vi "robust-battery-agent.vi"() -> ()   [LabVIEW 2021]
uses:
  General purpose/MEAS.ctl
  General purpose/REQ.ctl
  General purpose/agent-variables.ctl
  General purpose/daemon-config.ctl
panel:
  in  "daemon-config":T1={"resource-type"="battery", "agent-id"=12, "GA-ip"="192.168.1.1", "GA-port"=52020, "RA-ip"="127.0.0.1", "RA-port"=52001, "listenport-RA-side"=52011, "listenport-GA-side"=52021, "local-ip"="192.168.1.12", "long-term"=FALSE}
  in  "param":T2={"Srated"=25000.0, "eta [pu]"=0.98, "model"={"in-states"={"v1"=0.0, "v2"=0.0, "SoC"=0.0}, "output"={"V"=0.0, "Zeq"=0.0, "Eeq"=0.0}}} {"model"."output"."Eeq" format="%#.6g"; "model"."output"."Zeq" format="%#.6g"; "eta [pu]" format="%#_13g"}
  out "json-adv":string
  out "error out":errorcluster
  in  "ra-res config":T3={"resource-type"="battery", "res-ip"="127.0.0.1", "write-port"=32001, "listen-port"=32011}
  out "wake-up":timestamp
  out "uc":cluster{"Pc":dbl, "Qc":dbl}
  in  "model-dt":u32=100
  in  "SoC_T":dbl=50.0
  out "REQ":T4
  in  "main stop":bool
  out "Meas":T5 {"Ud" format="%#.2f"; "P" format="%#.2f"; "Q" format="%#.2f"}
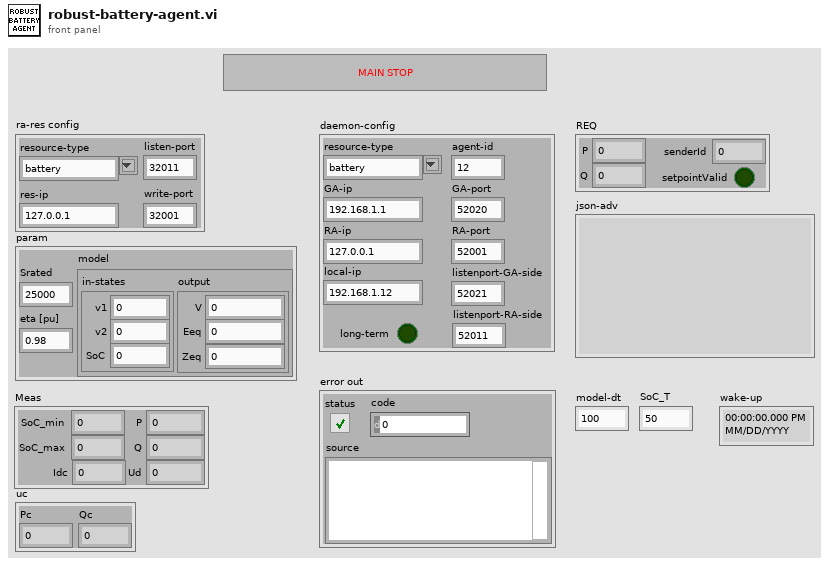
[diagram p1: front panel]
types:
  T1 = typedef "daemon-config.ctl" = cluster{"resource-type":string, "agent-id":u16, "GA-ip":string, "GA-port":u16, "RA-ip":string, "RA-port":u16, "listenport-RA-side":u16, "listenport-GA-side":u16, "local-ip":string, "long-term":bool}
  T2 = typedef "agent-variables.ctl" = cluster{"Srated":dbl, "eta [pu]":dbl, "model":cluster{"in-states":cluster{"v1":dbl, "v2":dbl, "SoC":dbl}, "output":cluster{"V":dbl, "Zeq":dbl, "Eeq":dbl}}}
  T3 = cluster{"resource-type":string, "res-ip":string, "write-port":u16, "listen-port":u16}
  T4 = typedef "REQ.ctl" = cluster{"P":dbl, "Q":dbl, "senderId":u32, "setpointValid":bool}
  T5 = typedef "MEAS.ctl" = cluster{"P":dbl, "Q":dbl, "SoC_max":dbl, "SoC_min":dbl, "Ud":dbl, "Idc":dbl}
  T6 = cluster{"in-states":cluster{"v1":dbl, "v2":dbl, "SoC":dbl}, "output":cluster{"V":dbl, "Zeq":dbl, "Eeq":dbl}}
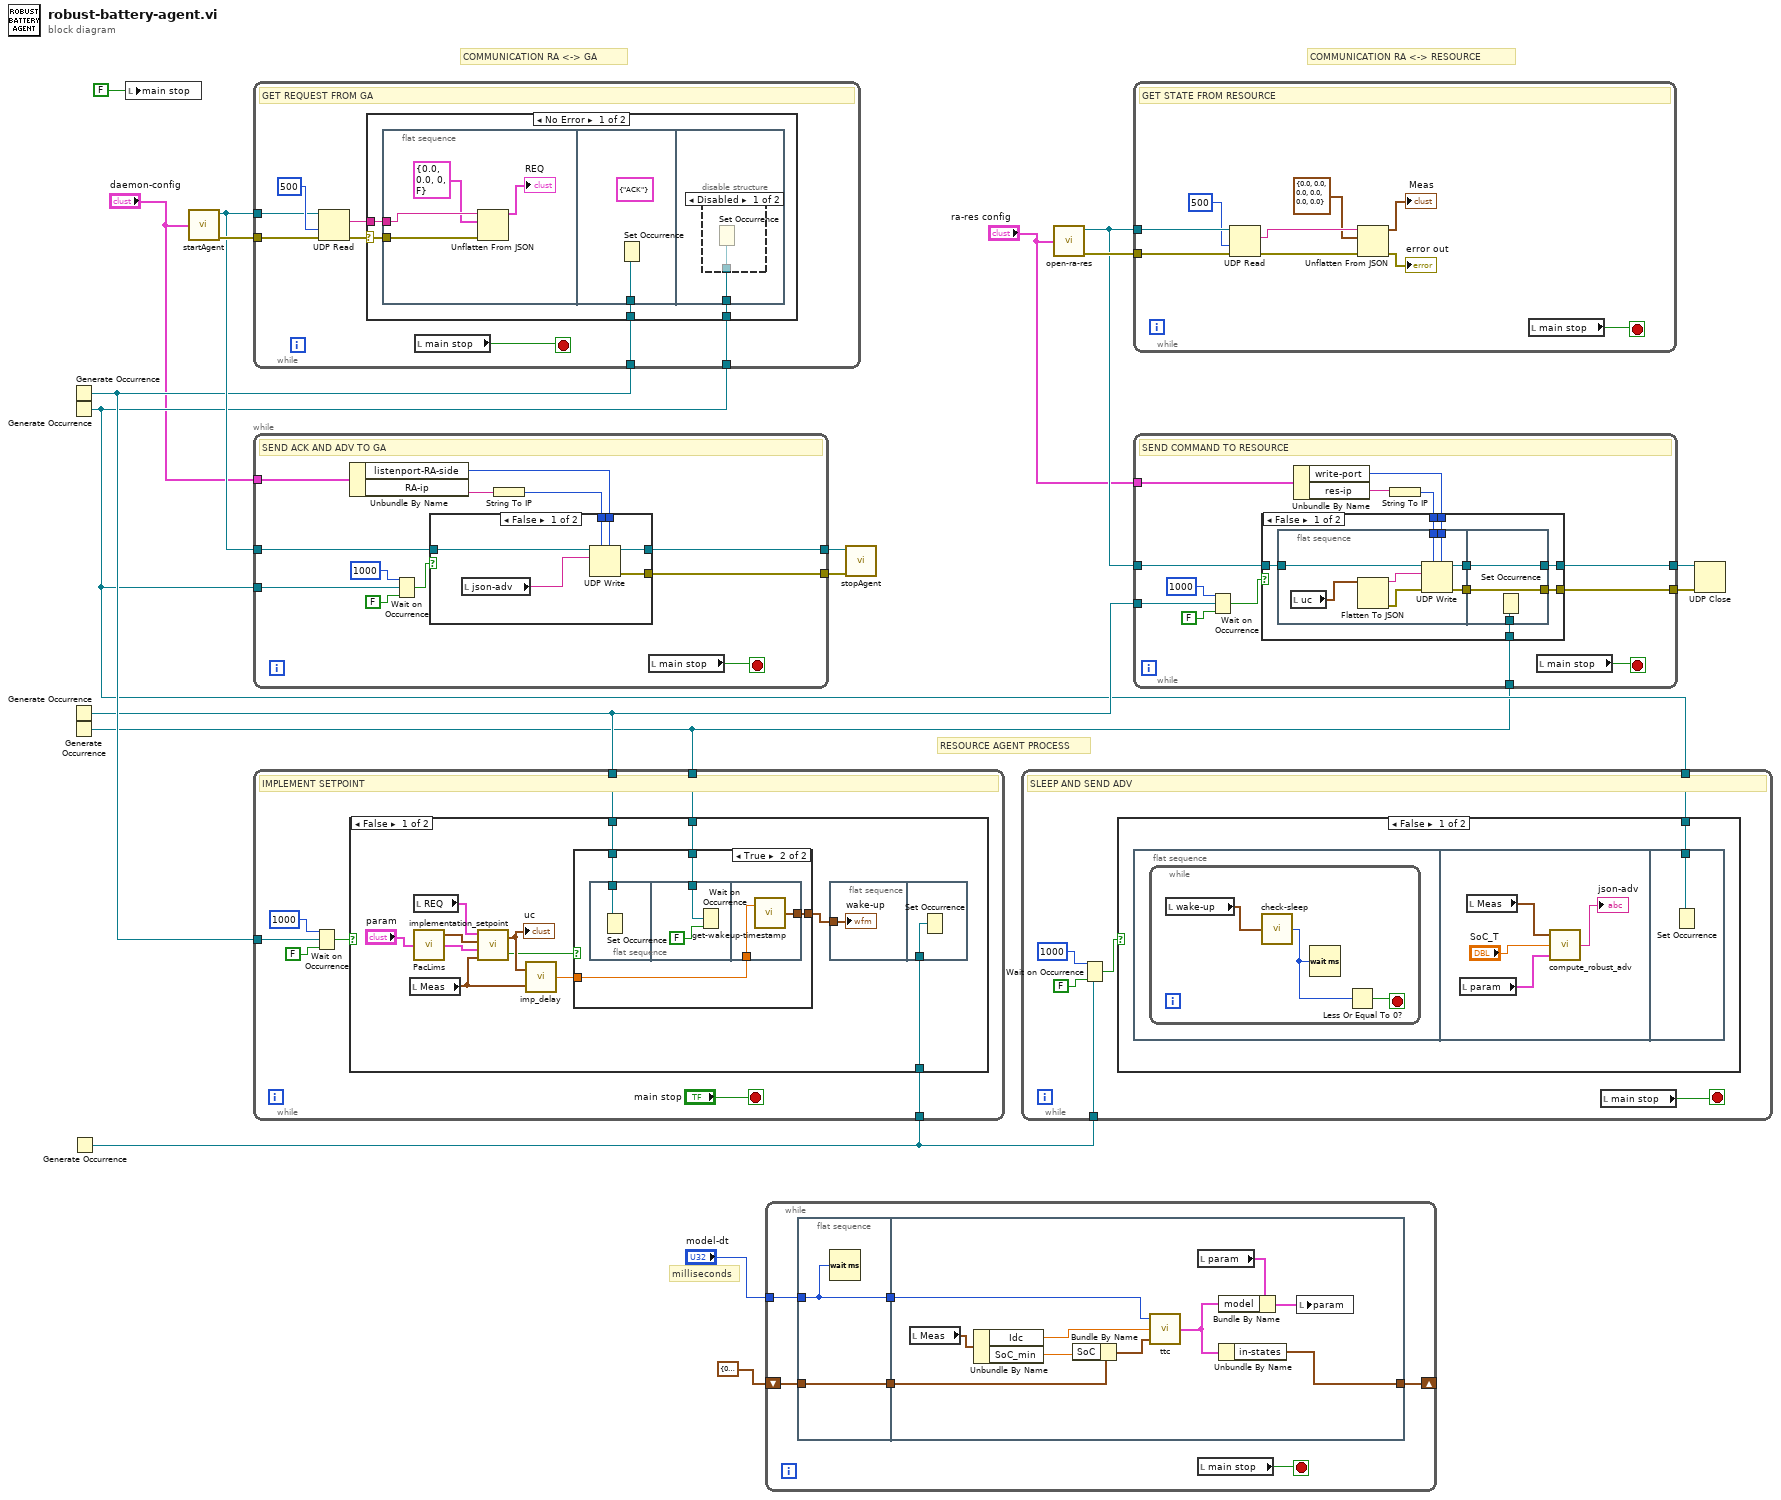
[diagram p0: block diagram]
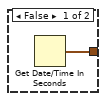
[diagram p2: hidden frame]
diagram:
  # "milliseconds"
  # "RESOURCE AGENT PROCESS"
  # "COMMUNICATION RA <-> RESOURCE"
  # "COMMUNICATION RA <-> GA"
  n1 = Generate Occurrence() -> (w14:refnum<k4>)
  n2 = Generate Occurrence() -> (w12:refnum<k4>)
  n3 = Generate Occurrence() -> (w13:refnum<k4>)
  n4 = Generate Occurrence() -> (w11:refnum<k4>)
  n5 = Generate Occurrence() -> (w4:refnum<k4>)
  n6 = local write "main stop"(FALSE ("main stop")) -> ()
  n7 = call "startAgent.vi"("daemon-config"="daemon-config") -> ("error out"=w18:errorcluster, "connection ID"=w15:refnum<k16>)  [unwired: 6 in]
  n8 = while {
    tunnel: w15 -> [w22]
    tunnel: w18 -> [w21]
    tunnel: w14 -> [w25]
    tunnel: w12 -> [w24]
    stop <- w26 stop-if-true
    # "GET REQUEST FROM GA"
    n9 = UDP Read(connection ID=w22, timeout ms (25000)=500, 8:w21) -> (data out=w19:string, error out=w20:errorcluster)  [unwired: 4 out]
    n10 = case shown="No Error" w20 {
      selector: w20 -> [w28 _]
      tunnel: w25 -> [w30 _]
      tunnel: w24 -> [w29 _]
      tunnel: w19 -> [w27 _]
      frame No Error {
        n11 = flat-sequence {
          tunnel: w28 -> [w33]
          tunnel: w27 -> [w32]
          tunnel: w30 -> [w35]
          tunnel: w29 -> [w36]
          frame #0 {
            n12 = Unflatten From JSON(JSON string=w32, type and defaults=T4 {"P"=0.0, "Q"=0.0, "senderId"=0, "setpointValid"=FALSE} ("REQ"), error in (no error)=w33) -> (value=→"REQ":T4)  [unwired: 4 in, 1 out]
          }
          frame #1 {
            (unwired) cluster{string} {"ACK"} ("anything")
            n13 = Set Occurrence(w35) -> ()
          }
          frame #2 {
            n14 = disable-structure shown="Disabled" {
              disable-tunnel: w36 -> [w37 _]
              frame Disabled {
                n15 = Set Occurrence(w37) -> ()
              }
              frame Enabled {
              }
            }
          }
        }
      }
      frame Error {
      }
    }
    n16 = local read "main stop"() -> (w26:bool)
  }
  n17 = while {
    tunnel: [w48] -> w17
    tunnel: [w47] -> w16
    tunnel: "daemon-config" -> [w45]
    tunnel: w12 -> [w42]
    tunnel: w15 -> [w41]
    stop <- w49 stop-if-true
    # "SEND ACK AND ADV TO GA"
    n18 = Unbundle By Name(w45) -> ("listenport-RA-side"=w43:u16, "RA-ip"=w46:string)
    n19 = Wait on Occurrence(1:FALSE ("ignore previous (T)"), 2:w42, 3:1000 ("ms timeout (-1)")) -> (0:w40:bool)
    n20 = String To IP(1:w46) -> (0:w44:u32)
    n21 = case shown="False" w40 {
      tunnel: [w55 w56] -> w48
      tunnel: [w54 _] -> w47
      tunnel: w44 -> [w53 _]
      tunnel: w43 -> [w52 _]
      tunnel: w41 -> [w51 w56]
      frame False {
        n22 = local read "json-adv"() -> (w50:string)
        n23 = UDP Write(address=w53, port or service name=w52, connection ID=w51, data in=w50) -> (error out=w54:errorcluster, 3:w55:refnum<k16>)  [unwired: 2 in]
      }
      frame True {
      }
    }
    n24 = local read "main stop"() -> (w49:bool)
  }
  n25 = while {
    tunnel: w14 -> [w58]
    tunnel: w13 -> [w64]
    tunnel: w11 -> [w62]
    tunnel: w4 -> [w61]
    stop <- "main stop" stop-if-true
    # "IMPLEMENT SETPOINT"
    n26 = Wait on Occurrence(1:FALSE ("ignore previous (T)"), 2:w58, 3:1000 ("ms timeout (-1)")) -> (0:w60:bool)
    n27 = case shown="False" w60 {
      tunnel: w64 -> [w76 _]
      tunnel: w62 -> [w75 _]
      tunnel: w61 -> [w66 _]
      frame False {
        n28 = local read "Meas"() -> (w70:T5)
        n29 = local read "REQ"() -> (w72:T4)
        n30 = call "PacLims.vi"("param (in)"="param") -> ("PacLims"=w74:cluster{"Pmax":dbl, "Pmin":dbl}, "param (out)"=w73:T2)  [unwired: 1 out]
        n31 = call "implementation_setpoint.vi"("Meas"=w70, "param"=w73, "PacLims (in)"=w74, "REQ"=w72) -> ("send_cmd?"=w69:bool, "uc"=w71:cluster{"Pc":dbl, "Qc":dbl})
        "uc" <- w71
        n32 = call "imp_delay.vi"("Meas"=w70, "uc"=w71) -> ("res-dt"=w68:dbl)
        n33 = case shown="True" w69 {
          tunnel: w76 -> [_ w83]
          tunnel: w75 -> [_ w82]
          tunnel: w68 -> [_ w81]
          tunnel: [w79 w80] -> w67
          frame False {
            n34 = Get Date/Time In Seconds() -> (seconds since 1Jan1904=w79:timestamp)
          }
          frame True {
            n35 = flat-sequence {
              tunnel: w83 -> [w84]
              tunnel: w82 -> [w86]
              tunnel: w81 -> [w88]
              tunnel: [w87] -> w80
              frame #0 {
                n36 = Set Occurrence(w84) -> ()
              }
              frame #1 {
                n37 = Wait on Occurrence(1:FALSE ("ignore previous (T)"), 2:w86) -> ()  [unwired: 1 in, 1 out]
              }
              frame #2 {
                n38 = call "get-wakeup-timestamp.vi"("Tra"=w88) -> ("wake-up timestamp"=w87:timestamp)  [unwired: 1 in]
              }
            }
          }
        }
        n39 = flat-sequence {
          tunnel: w67 -> [w77]
          tunnel: w66 -> [w78]
          frame #0 {
            "wake-up" <- w77
          }
          frame #1 {
            n40 = Set Occurrence(w78) -> ()
          }
        }
      }
      frame True {
      }
    }
  }
  n41 = while {
    tunnel: "model-dt" -> [w93]
    shift-right: [w92] -> _
    shift-left: cluster{"v1":dbl, "v2":dbl, "SoC":dbl} {"v1"=0.0, "v2"=0.0, "SoC"=0.0} ("in-states") -> [w90]
    stop <- w94 stop-if-true
    n42 = flat-sequence {
      tunnel: w93 -> [w95]
      tunnel: [w96] -> w91
      tunnel: w90 -> [w96]
      tunnel: [w95] -> w89
      tunnel: [w103] -> w92
      tunnel: w91 -> [w101]
      tunnel: w89 -> [w97]
      frame #0 {
        n43 = Wait (ms)(milliseconds to wait=w95) -> ()  [unwired: 1 out]
      }
      frame #1 {
        n44 = local read "Meas"() -> (w106:T5)
        n45 = Unbundle By Name(w106) -> ("Idc"=w105:dbl, "SoC_min"=w99:dbl)
        n46 = Bundle By Name(cluster=w101, "SoC"=w99) -> (w100:cluster{"v1":dbl, "v2":dbl, "SoC":dbl})
        n47 = call "ttc.vi"("x[k-1]"=w100, "I"=w105, "Period"=w97) -> ("model"=w102:T6)  [unwired: 2 in]
        n48 = local read "param"() -> (w98:T2)
        n49 = Bundle By Name(cluster=w98, "model"=w102) -> (w104:T2)
        n50 = Unbundle By Name(w102) -> ("in-states"=w103:cluster{"v1":dbl, "v2":dbl, "SoC":dbl})
        n51 = local write "param"(w104) -> ()
      }
    }
    n52 = local read "main stop"() -> (w94:bool)
  }
  n53 = call "stopAgent.vi"("error in"=w16, "connection ID"=w17) -> ()  [unwired: 10 in]
  n54 = while {
    tunnel: w4 -> [w109]
    tunnel: w12 -> [w111]
    stop <- w112 stop-if-true
    # "SLEEP AND SEND ADV"
    n55 = Wait on Occurrence(1:FALSE ("ignore previous (T)"), 2:w109, 3:1000 ("ms timeout (-1)")) -> (0:w110:bool)
    n56 = case shown="False" w110 {
      tunnel: w111 -> [w113 _]
      frame False {
        n57 = flat-sequence {
          tunnel: w113 -> [w121]
          frame #0 {
            n58 = while {
              stop <- w115 stop-if-true
              n59 = local read "wake-up"() -> (w116:timestamp)
              n60 = call "check-sleep.vi"("wake-up timestamp"=w116) -> ("dt"=w114:u32)
              n61 = Wait (ms)(milliseconds to wait=w114) -> ()  [unwired: 1 out]
              n62 = Less Or Equal To 0?(x=w114) -> (x <= 0?=w115:bool)
            }
          }
          frame #1 {
            n63 = local read "param"() -> (w117:T2)
            n64 = local read "Meas"() -> (w120:T5)
            n65 = call "compute_robust_adv.vi"("param"=w117, "SoC_T"="SoC_T", "Meas"=w120) -> ("json-adv"=→"json-adv":string)
          }
          frame #2 {
            n66 = Set Occurrence(w121) -> ()
          }
        }
      }
      frame True {
      }
    }
    n67 = local read "main stop"() -> (w112:bool)
  }
  n68 = call "open-ra-res.vi"("config"="ra-res config") -> ("error out"=w10:errorcluster, "connection ID"=w9:refnum<k16>)  [unwired: 6 in]
  n69 = while {
    tunnel: w9 -> [w129]
    tunnel: w10 -> [w128]
    stop <- w130 stop-if-true
    # "GET STATE FROM RESOURCE"
    n70 = UDP Read(connection ID=w129, timeout ms (25000)=500, 8:w128) -> (data out=w126:string, error out=w125:errorcluster)  [unwired: 4 out]
    n71 = Unflatten From JSON(JSON string=w126, type and defaults=T5 {"P"=0.0, "Q"=0.0, "SoC_max"=0.0, "SoC_min"=0.0, "Ud"=0.0, "Idc"=0.0} ("Meas"), error in (no error)=w125) -> (value=→"Meas":T5, error out=→"error out":errorcluster)  [unwired: 4 in]
    n72 = local read "main stop"() -> (w130:bool)
  }
  n73 = while {
    tunnel: [w142] -> w8
    tunnel: [w141] -> w7
    tunnel: w13 -> [w135]
    tunnel: w9 -> [w140]
    tunnel: w11 -> [w132]
    tunnel: "ra-res config" -> [w139]
    stop <- w143 stop-if-true
    # "SEND COMMAND TO RESOURCE"
    n74 = Wait on Occurrence(1:FALSE ("ignore previous (T)"), 2:w135, 3:1000 ("ms timeout (-1)")) -> (0:w133:bool)
    n75 = Unbundle By Name(w139) -> ("write-port"=w136:u16, "res-ip"=w138:string)
    n76 = String To IP(1:w138) -> (0:w137:u32)
    n77 = case shown="False" w133 {
      tunnel: [w151 w163] -> w142
      tunnel: [w150 _] -> w141
      tunnel: w140 -> [w149 w163]
      tunnel: w137 -> [w148 _]
      tunnel: w136 -> [w147 _]
      tunnel: w132 -> [w144 _]
      frame False {
        n78 = flat-sequence {
          tunnel: w149 -> [w157]
          tunnel: w148 -> [w156]
          tunnel: w147 -> [w155]
          tunnel: [w159] -> w146
          tunnel: [w158] -> w145
          tunnel: [w161] -> w150
          tunnel: [w162] -> w151
          tunnel: w146 -> [w162]
          tunnel: w145 -> [w161]
          tunnel: w144 -> [w160]
          frame #0 {
            n79 = local read "uc"() -> (w152:cluster{"Pc":dbl, "Qc":dbl})
            n80 = Flatten To JSON(anything=w152) -> (JSON string=w153:string, 11:w154:errorcluster)  [unwired: 2 in]
            n81 = UDP Write(address=w156, port or service name=w155, connection ID=w157, data in=w153, 8:w154) -> (error out=w158:errorcluster, 3:w159:refnum<k16>)  [unwired: 1 in]
          }
          frame #1 {
            n82 = Set Occurrence(w160) -> ()
          }
        }
      }
      frame True {
      }
    }
    n83 = local read "main stop"() -> (w143:bool)
  }
  n84 = UDP Close(connection ID=w8, 8:w7) -> ()  [unwired: 2 out]
